vi "JKI.Robot.SMO.Main.SIM.vi"() -> ()   [LabVIEW 2015]
doc: "JKI State Machine Objects (SMO) 1.0.0.5\nJKI - JKI\nCopyright (c) 2016, JKI"
uses:
  JKI.Robot.SMO.TestUI/JKI.Robot.SMO.APITesterUI.lvclass
  JKI.Robot.SMO.lvclass
  JKI.Robot.SMO.TestUI/JKI.Robot.SMO.APITesterUI.lvclass/JKI.Robot.SMO.APITesterUI.ctl
  <vilib>/JKI/JKI SMO/SMO/SMO.lvclass
  <vilib>/JKI/JKI SMO/SMO.UI/SMO.UI.lvclass
panel:
  out "error out":errorcluster
  in  "Stop":bool
  # "BB9 APP LAUNCHER"
  # "For instructions on how to use the JKI State Machine Objects, examples and video tutorials, visit:\nhttp://jki.net/state-machine-objects/\n\nJKI State Machine Objects™\nhttp://jki.net/state-machine-objects/\nCopyright (C) 2005-2015, JKI <info@jki.net>\nALL RIGHTS RESERVED"
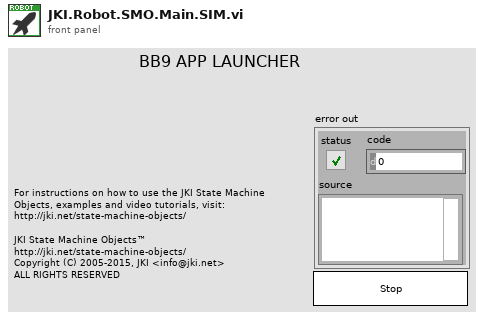
[diagram p1: front panel]
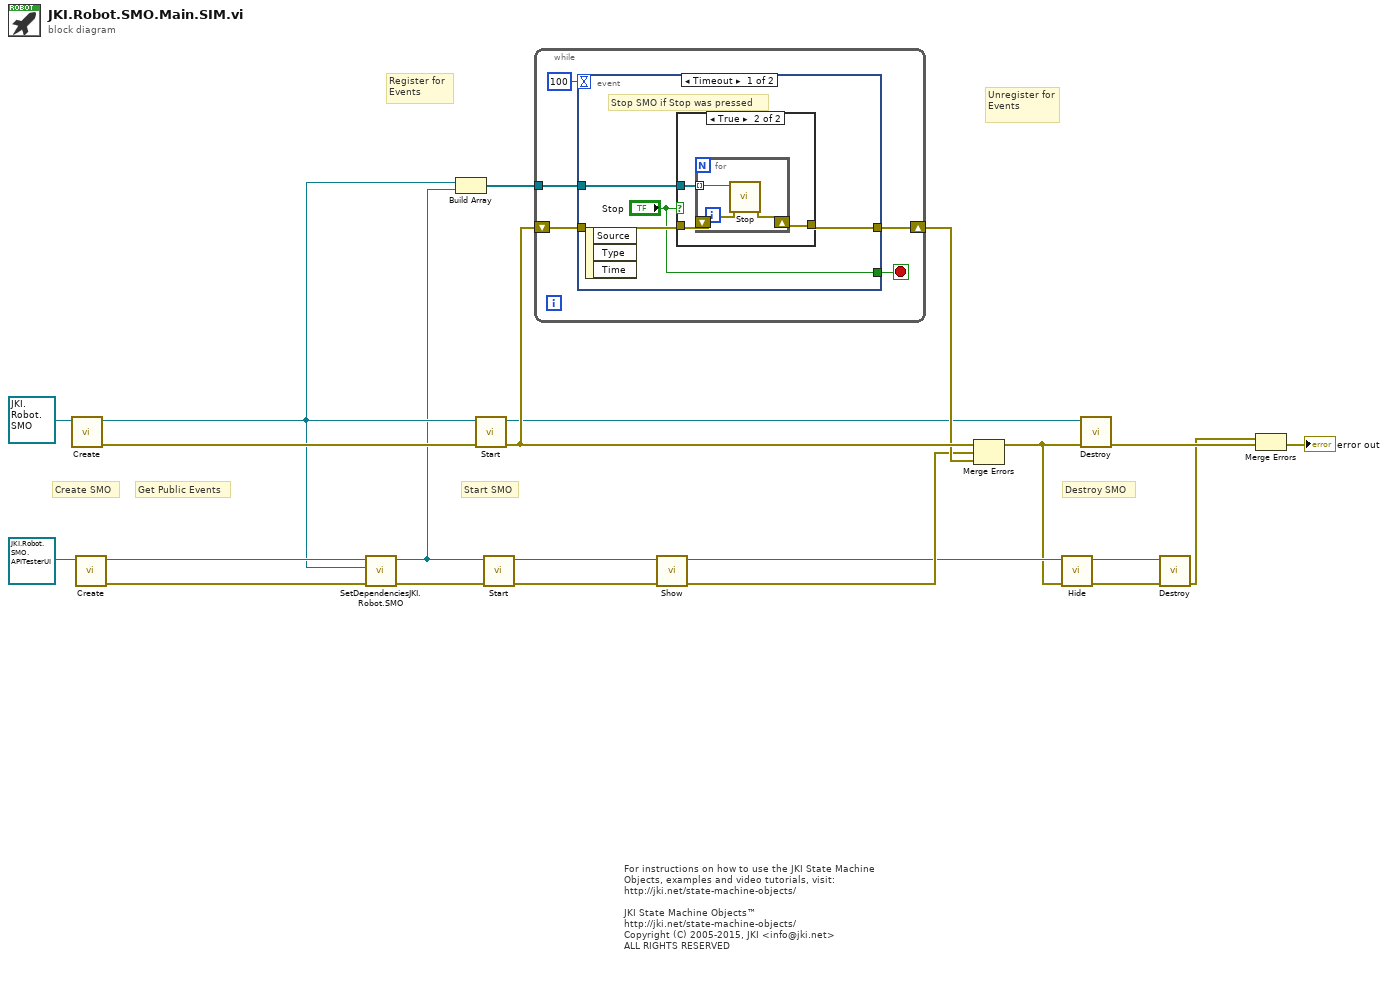
[diagram p0: block diagram]
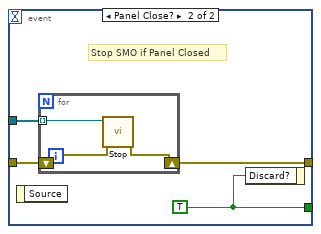
[diagram p3: hidden frame]
diagram:
  # "Get Public Events"
  # "Create SMO"
  # "Start SMO"
  # "Destroy SMO"
  # "For instructions on how to use the JKI State Machine Objects, examples and video tutorials, visit:\nhttp://jki.net/state-machine-objects/\n\nJKI State Machine Objects™\nhttp://jki.net/state-machine-objects/\nCopyright (C) 2005-2015, JKI <info@jki.net>\nALL RIGHTS RESERVED"
  # "Unregister for Events"
  # "Register for Events"
  n1 = call <vilib>:"Create.vi"("SMO"=refnum<class "JKI.Robot.SMO.lvclass"> refnum ("SMO.Template.lvclass")) -> ("error out"=w8:errorcluster, "SMO out"=w5:refnum<class "JKI.Robot.SMO.lvclass">)  [unwired: 8 in, 1 out]
  n2 = call <vilib>:"Create.vi"("SMO"=refnum<class "JKI.Robot.SMO.APITesterUI.lvclass"> refnum ("JKI.Robot.SMO.APITesterUI.lvclass")) -> ("error out"=w9:errorcluster, "SMO out"=w10:refnum<class "JKI.Robot.SMO.APITesterUI.lvclass">)  [unwired: 8 in, 1 out]
  n3 = call "SetDependenciesJKI.Robot.SMO.vi"("error in (no error)"=w9, "JKI.Robot"=w5, "JKI.Robot.SMO.APITesterUI in"=w10) -> ("error out"=w19:errorcluster, "JKI.Robot.SMO.APITesterUI out"=w4:refnum<class "JKI.Robot.SMO.APITesterUI.lvclass">)  [unwired: 7 in]
  n4 = Build Array(w5, w4) -> (w3:refnum<class "SMO.lvclass">[])
  n5 = call <vilib>:"Start.vi"("error in (no error)"=w8, "SMO"=w5) -> ("error out"=w20:errorcluster, "SMO out"=w7:refnum<class "JKI.Robot.SMO.lvclass">)  [unwired: 8 in]
  n6 = call <vilib>:"Start.vi"("error in (no error)"=w19, "SMO"=w4) -> ("error out"=w16:errorcluster, "SMO out"=w17:refnum<class "JKI.Robot.SMO.APITesterUI.lvclass">)  [unwired: 8 in]
  n7 = while {
    shift-right: [w26] -> w18
    shift-left: w20 -> [w25]
    tunnel: w3 -> [w23]
    stop <- w27 stop-if-true
    n8 = event shown="[0] Timeout" {
      selector: _ -> [_ _]
      dyn-events: _ -> [_ _]
      timeout: 100 -> [_ _]
      tunnel: ["Stop" w40] -> w27
      tunnel: [w31 w42] -> w26
      tunnel: w25 -> [w30 w41]
      tunnel: w23 -> [w28 w39]
      event Timeout {
        # "Stop SMO if Stop was pressed"
        n9 = event-data() -> ()  [unwired: 1 in, 3 out]
        n10 = case shown="True" "Stop" {
          tunnel: [w32 w35] -> w31
          tunnel: w30 -> [w32 w34]
          tunnel: w28 -> [_ w33]
          frame False {
          }
          frame True {
            n11 = for {
              shift-right: [w38] -> w35
              shift-left: w34 -> [w37]
              tunnel: w33 -> [w36] mode=indexing
              n12 = call <vilib>:"Stop.vi"("error in (no error)"=w37, "SMO"=w36) -> ("error out"=w38:errorcluster)  [unwired: 8 in, 1 out]
            }
          }
        }
      }
      event Panel Close? {
        w40 = TRUE ("OK")
        # "Stop SMO if Panel Closed"
        n13 = event-data() -> ()  [unwired: 1 in, 1 out]
        n14 = for {
          shift-right: [w45] -> w42
          shift-left: w41 -> [w44]
          tunnel: w39 -> [w43] mode=indexing
          n15 = call <vilib>:"Stop.vi"("error in (no error)"=w44, "SMO"=w43) -> ("error out"=w45:errorcluster)  [unwired: 8 in, 1 out]
        }
        n16 = event-data("Discard?"=w40) -> ()  [unwired: 1 in, 1 out]
      }
    }
  }
  n17 = call <vilib>:"Show.vi"("error in (no error)"=w16, "SMO.UI"=w17) -> ("error out"=w15:errorcluster, "SMO.UI out"=w14:refnum<class "JKI.Robot.SMO.APITesterUI.lvclass">)  [unwired: 8 in]
  n18 = Merge Errors(w20, w15, w18) -> (w2:errorcluster)
  n19 = call <vilib>:"Hide.vi"("error in (no error)"=w2, "SMO.UI"=w14) -> ("error out"=w12:errorcluster, "SMO.UI out"=w13:refnum<class "JKI.Robot.SMO.APITesterUI.lvclass">)  [unwired: 8 in]
  n20 = call <vilib>:"Destroy.vi"("error in (no error)"=w2, "SMO"=w7) -> ("error out"=w21:errorcluster)  [unwired: 9 in]
  n21 = call <vilib>:"Destroy.vi"("error in (no error)"=w12, "SMO"=w13) -> ("error out"=w6:errorcluster)  [unwired: 9 in]
  n22 = Merge Errors(w6, w21) -> (→"error out":errorcluster)
